vi "Write age using variant.vi"(10 "age":dbl, 11 "variant in":variant) -> (2 "error out":errorcluster, 3 "variant out":variant)   [LabVIEW 2012]
uses:
  ClassDefinitions/SimpleClassWithProperties/myClass.lvclass
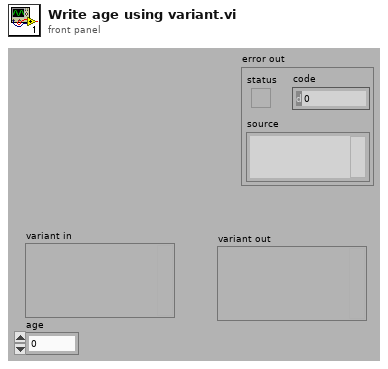
[diagram p1: front panel]
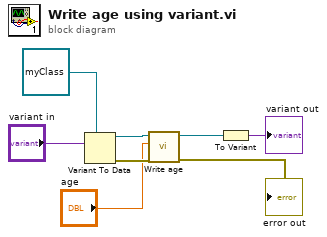
[diagram p0: block diagram]
diagram:
  n1 = Variant To Data(type=refnum<class "myClass.lvclass"> refnum ("myClass.lvclass"), Variant="variant in") -> (data=w5:refnum<class "myClass.lvclass">, error out=w4:errorcluster)  [unwired: 1 in]
  n2 = call-dynamic "Write age.vi"("error in (no error)"=w4, "age"="age", "myClass in"=w5) -> ("error out"=→"error out":errorcluster, "myClass out"=w2:refnum<class "myClass.lvclass">)  [unwired: 7 in]
  n3 = To Variant(anything=w2) -> (Variant=→"variant out":variant)
